vi "Scan Insert Type.vi"(10 "Lookup Path":path) -> (0 "OK?":bool, 2 "Insert Type Out":string)   [LabVIEW 2026]
panel:
  out "First Scan?":bool
  in  "Case Constant\n(See Context Help)":bool
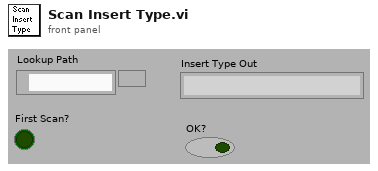
[diagram p1: front panel]
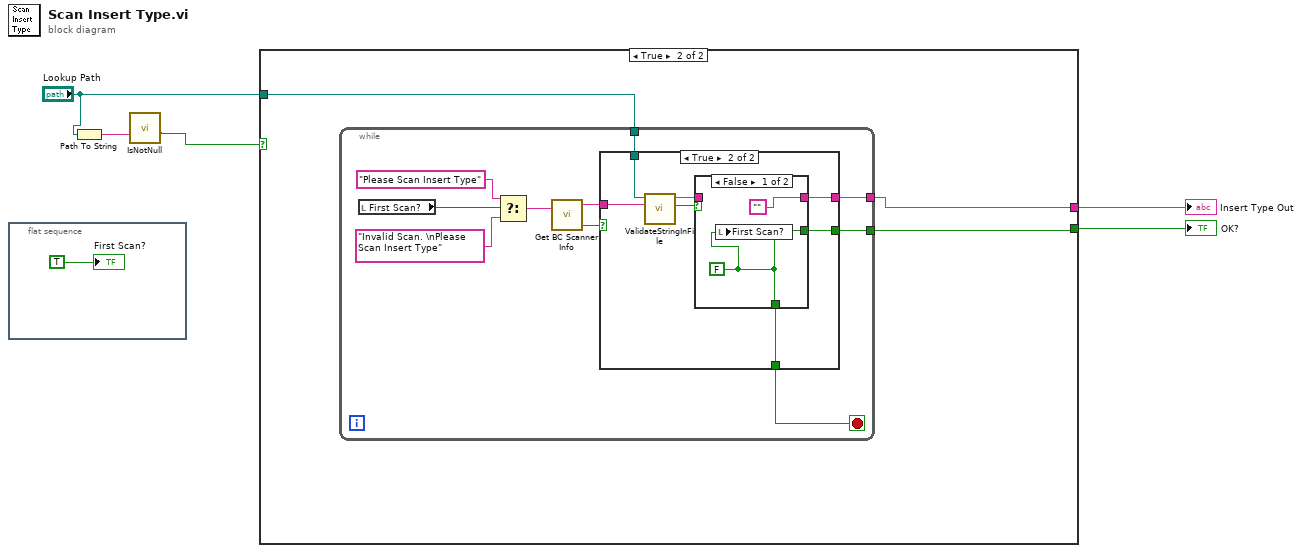
[diagram p0: block diagram]
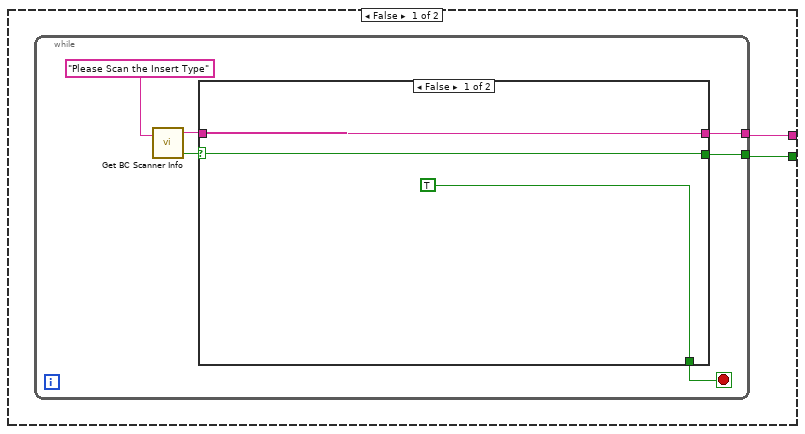
[diagram p2: hidden frame]
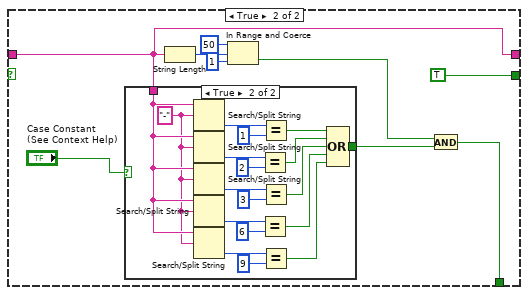
[diagram p3: hidden frame]
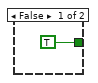
[diagram p4: hidden frame]
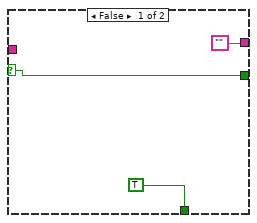
[diagram p5: hidden frame]
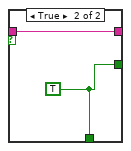
[diagram p6: hidden frame]
diagram:
  n1 = flat-sequence {
    frame #0 {
      "First Scan?" <- TRUE
    }
  }
  n2 = Path To String(path="Lookup Path") -> (string=w2:string)
  n3 = call "IsNotNull.vi"("String In"=w2) -> ("Boolean Out"=w1:bool)  [unwired: 10 in]
  n4 = case shown="True" w1 {
    tunnel: [w8 w47] -> w5
    tunnel: [w7 w46] -> w4
    tunnel: "Lookup Path" -> [_ w48]
    frame False {
      n5 = while {
        tunnel: [w9] -> w7
        tunnel: [w11] -> w8
        stop <- w10 stop-if-true
        n6 = call "Get BC Scanner Info.vi"("Prompt"="Please Scan the Insert Type") -> ("Info Out"=w12:string, "OK"=w13:bool)  [unwired: 2 in]
        n7 = case shown="False" w13 {
          selector: w13 -> [w15 _]
          tunnel: w12 -> [w17 w22]
          tunnel: [w17 w22] -> w11
          tunnel: [TRUE ("OK") w21] -> w10
          tunnel: [w15 TRUE ("OK")] -> w9
          frame False {
          }
          frame True {
            n8 = case shown="True" "Case Constant\n(See Context Help)" {
              tunnel: w22 -> [_ w35]
              tunnel: [TRUE w28] -> w20
              frame False {
              }
              frame True {
                w34 = "-" ("search string/char (-)")
                n9 = Search/Split String(string=w35, search string/char (-)=w34) -> (offset of match=w45:i32)  [unwired: 1 in, 2 out]
                n10 = Search/Split String(string=w35, search string/char (-)=w34) -> (offset of match=w44:i32)  [unwired: 1 in, 2 out]
                n11 = Search/Split String(string=w35, search string/char (-)=w34) -> (offset of match=w38:i32)  [unwired: 1 in, 2 out]
                n12 = Search/Split String(string=w35, search string/char (-)=w34) -> (offset of match=w39:i32)  [unwired: 1 in, 2 out]
                n13 = Search/Split String(string=w35, search string/char (-)=w34) -> (offset of match=w37:i32)  [unwired: 1 in, 2 out]
                n14 = Equal?(x=w44, y=2) -> (x = y?=w32:bool)
                n15 = Equal?(x=w39, y=6) -> (x = y?=w30:bool)
                n16 = Equal?(x=w45, y=1) -> (x = y?=w33:bool)
                n17 = Equal?(x=w38, y=3) -> (x = y?=w31:bool)
                n18 = Equal?(x=w37, y=9) -> (x = y?=w29:bool)
                n19 = Compound Arithmetic op=OR(w33, w32, w31, w30, w29) -> (w28:bool)
              }
            }
            n20 = String Length(string=w22) -> (length=w25:i32)
            n21 = In Range and Coerce(upper limit=50, x=w25, lower limit=1) -> (In Range?=w19:bool)  [unwired: 1 out]
            n22 = And(x=w19, y=w20) -> (x .and. y?=w21:bool)
          }
        }
      }
    }
    frame True {
      n23 = while {
        tunnel: w48 -> [w52]
        tunnel: [w51] -> w47
        tunnel: [w50] -> w46
        stop <- w49 stop-if-true
        n24 = local read "First Scan?"() -> (w56:bool)
        n25 = Select(t="Please Scan Insert Type", s=w56, f="Invalid Scan. \nPlease Scan Insert Type") -> (s? t:f=w55:string)
        n26 = call "Get BC Scanner Info.vi"("Prompt"=w55) -> ("Info Out"=w53:string, "OK"=w54:bool)  [unwired: 2 in]
        n27 = case shown="True" w54 {
          selector: w54 -> [w60 _]
          tunnel: w53 -> [_ w68]
          tunnel: w52 -> [_ w67]
          tunnel: ["" w64] -> w51
          tunnel: [w60 w63] -> w50
          tunnel: [TRUE w62] -> w49
          frame False {
          }
          frame True {
            n28 = call "ValidateStringInFile.vi"("String to find"=w68, "Path In"=w67) -> ("String Found"=w66:bool, "String Out"=w65:string)  [unwired: 7 in, 1 out]
            n29 = case shown="False" w66 {
              tunnel: w65 -> [_ w72]
              tunnel: ["" w72] -> w64
              tunnel: [w70 w71] -> w63
              tunnel: [w70 w71] -> w62
              frame False {
                w70 = FALSE
                n30 = local write "First Scan?"(w70) -> ()
              }
              frame True {
                w71 = TRUE
              }
            }
          }
        }
      }
    }
  }
  "Insert Type Out" <- w5
  "OK?" <- w4
